vi "GetCluster.vi"(8 "error in (no error)":errorcluster, 11 "syslogs in":refnum<class "syslogs.lvclass">) -> (0 "error out":errorcluster, 2 "Value":T1={"id"=0, "type"="info", "executiontime"=0.0, "log"="", "guid"="", "Time Stamp"=timestamp(0 s since 1904-01-01)} {"Time Stamp" format="%<%x %.3X>T"}, 3 "syslogs out":refnum<class "syslogs.lvclass">)   [LabVIEW 2020, in "ORM_Examples.lvlib" / "syslogs.lvclass"]
uses:
  syslogs.lvclass
  syslogcluster.ctl
  type.ctl
  syslogs.lvclass/syslogs.ctl
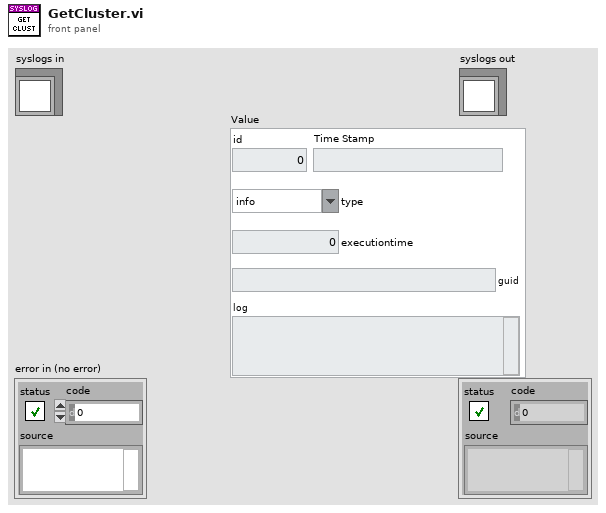
[diagram p1: front panel]
types:
  T1 = typedef "ORM_Examples.lvlib/syslogs.lvclass/syslogcluster.ctl" = cluster{"id":i32, "type":T2, "executiontime":dbl, "log":string, "guid":string, "Time Stamp":timestamp}
  T2 = typedef "ORM_Examples.lvlib/syslogs.lvclass/type.ctl" = string
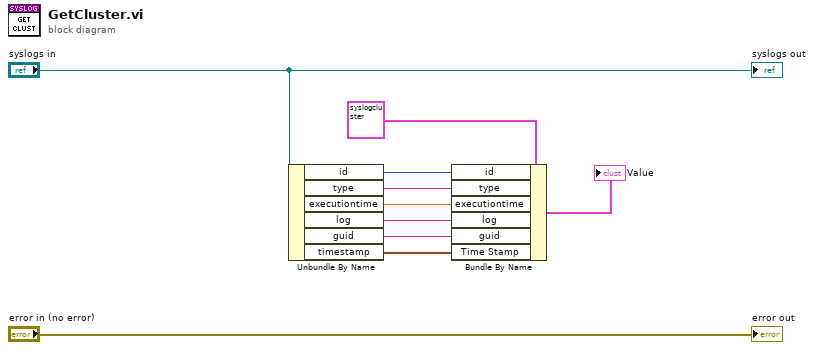
[diagram p0: block diagram]
diagram:
  n1 = Unbundle By Name("syslogs in") -> ("id"=w6:i32, "type"=w5:T2, "executiontime"=w4:dbl, "log"=w3:string, "guid"=w2:string, "timestamp"=w1:timestamp)
  n2 = Bundle By Name(cluster=T1 {"id"=0, "type"="info", "executiontime"=0.0, "log"="", "guid"="", "Time Stamp"=timestamp(0 s since 1904-01-01)} ("Cluster of class private data"), "id"=w6, "type"=w5, "executiontime"=w4, "log"=w3, "guid"=w2, "Time Stamp"=w1) -> (→"Value":T1)
  "error out" <- "error in (no error)"
  "syslogs out" <- "syslogs in"
